vi "Local Error Handler.vi"(7 "Default Action":T1, 8 "error in (no error)":errorcluster, 9 "Shutdown":i32[](array[numeric]), 10 "Log":i32[](array[numeric]), 11 "Ignore":i32[](array[numeric])) -> (0 "error out":errorcluster, 3 "Stop":bool)   [LabVIEW 2011]
uses:
  FPGA Control cRIO Demo Box/FPGA Control Template/Shared/Error Handler/Error Actions.ctl
  FPGA Control cRIO Demo Box/FPGA Control Template/Shared/Error Handler/Stop Method.ctl
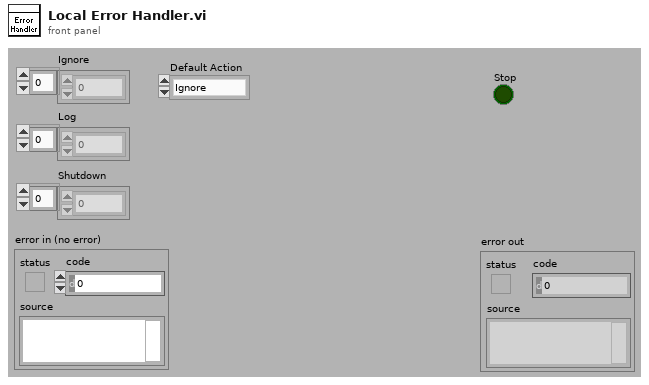
[diagram p1: front panel]
types:
  T1 = typedef "Error Actions.ctl" = enum16{"Ignore", "Log", "Shutdown"}
  T2 = typedef "Stop Method.ctl" = enum16{"Get", "Set"}
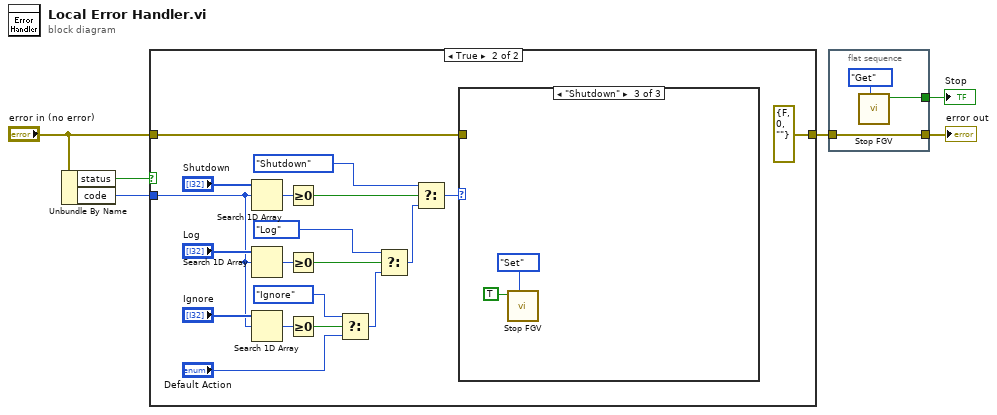
[diagram p0: block diagram]
diagram:
  n1 = Unbundle By Name("error in (no error)") -> ("status"=w6:bool, "code"=w5:i32)
  n2 = case shown="True" w6 {
    tunnel: w5 -> [_ w20]
    tunnel: "error in (no error)" -> [w7 w9]
    tunnel: [w7 errorcluster {"status"=FALSE, "code"=0, "source"=""} ("error out")] -> w3
    frame False {
    }
    frame True {
      n3 = Search 1D Array(1D array="Shutdown", element=w20) -> (index of element=w22:i32)  [unwired: 1 in]
      n4 = Search 1D Array(1D array="Log", element=w20) -> (index of element=w24:i32)  [unwired: 1 in]
      n5 = Search 1D Array(1D array="Ignore", element=w20) -> (index of element=w25:i32)  [unwired: 1 in]
      n6 = Greater Or Equal To 0?(x=w22) -> (x >= 0?=w13:bool)
      n7 = Greater Or Equal To 0?(x=w24) -> (x >= 0?=w16:bool)
      n8 = Greater Or Equal To 0?(x=w25) -> (x >= 0?=w18:bool)
      n9 = Select(t=Error_Actions."Ignore", s=w18, f="Default Action") -> (s? t:f=w15:T1)
      n10 = Select(t=Error_Actions."Log", s=w16, f=w15) -> (s? t:f=w12:T1)
      n11 = Select(t=Error_Actions."Shutdown", s=w13, f=w12) -> (s? t:f=w10:T1)
      n12 = case shown="\"Ignore\", Default" w10 {
        tunnel: w9 -> [_ _ _]
        frame "Ignore", Default {
        }
        frame "Log" {
        }
        frame "Shutdown" {
          n13 = call "Stop FGV.vi"("Method"=Stop_Method."Set", "Value"=TRUE) -> ()  [unwired: 9 in, 1 out]
        }
      }
    }
  }
  n14 = flat-sequence {
    tunnel: w3 -> [w30]
    tunnel: [w30] -> w2
    tunnel: [w29] -> w1
    frame #0 {
      n15 = call "Stop FGV.vi"("Method"=Stop_Method."Get") -> ("Stop"=w29:bool)  [unwired: 10 in]
    }
  }
  "error out" <- w2
  "Stop" <- w1
